vi "RT Init.vi"(8 "error in":errorcluster, 10 "Input Channels":T5[](array[typedef]) format="%.0x", 11 "Custom Device Ref in":T5 format="%.0x") -> (0 "error out":errorcluster, 3 "RT Configuration Data":T1 {"Cal Types" items=["J", "K", "T", "E", "N", "B", "R", "S"]; "Temperature Units" items=["Celcius", "Fahrenheit", "Kelvin", "Rankine"]; "TC Channel Config"."Temperature Units" items=["Celcius", "Fahrenheit", "Kelvin", "Rankine", "Volts"]; "TC Channel Config"."Thermocouple Type" items=["J", "K", "T", "E", "N", "B", "R", "S", "Raw Voltage"]})   [LabVIEW 2011, in "Simulated Thermocouple Custom Device.lvlib"]
uses:
  Simulated Thermocouple Custom Device.lvlib
  <vilib>/NI Veristand/Custom Device API/Custom Device Item Ref.ctl
  RT Config Data.ctl
  TC Channel Config Data.ctl
  TC Selector.ctl
  TC Unit Selector.ctl
  Device Settings.ctl
  Calibration Config Data.ctl
  VO Channel Config Data.ctl
  <vilib>/NI Veristand/Custom Device API/Get Item Property (Variant).vi
  <vilib>/NI Veristand/Custom Device API/Get Item Property (String).vi
  <vilib>/DAQmx/create/channels.llb/DAQmx Create Channel (AO-Voltage-Basic).vi
  <vilib>/DAQmx/create/channels.llb/DAQmx Create Channel (AO-Current-Basic).vi
  <vilib>/NI Veristand/Custom Device API/Custom Device API.lvlib
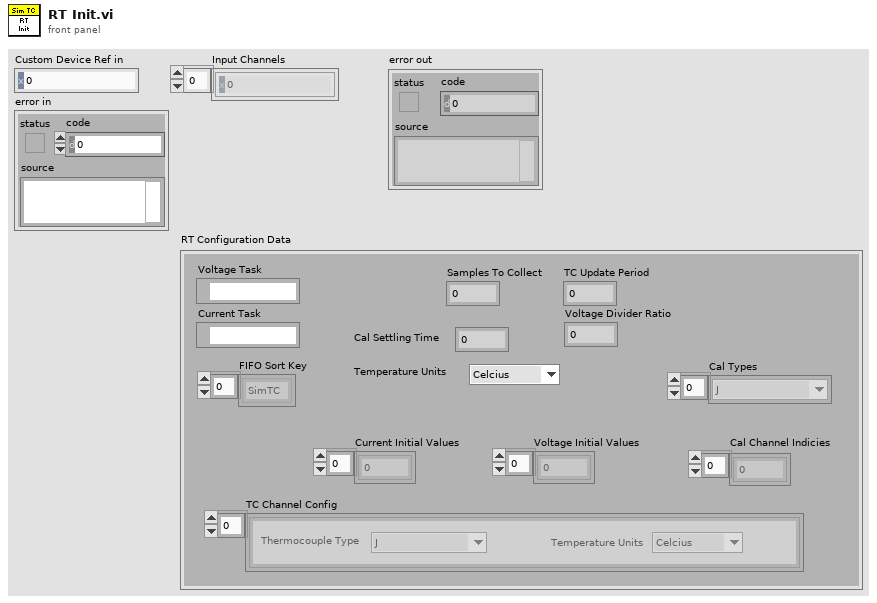
[diagram p1: front panel]
types:
  T1 = typedef "Simulated Thermocouple Custom Device.lvlib/RT Config Data.ctl" = cluster{"Current Task":refnum<k21>, "Voltage Task":refnum<k21>, "FIFO Sort Key":enum16{"SimTC", "Calibration", "VO", "CO"}[], "Cal Channel Indicies":i32[], "Current Initial Values":dbl[], "Voltage Initial Values":dbl[], "TC Channel Config":T2[], "TC Update Period":dbl, "Voltage Divider Ratio":dbl, "Samples To Collect":dbl, "Temperature Units":T4, "Cal Settling Time":dbl, "Cal Types":T3[]}
  T2 = typedef "Simulated Thermocouple Custom Device.lvlib/TC Channel Config Data.ctl" = cluster{"Thermocouple Type":T3, "Temperature Units":T4}
  T3 = typedef "Simulated Thermocouple Custom Device.lvlib/TC Selector.ctl" = u16
  T4 = typedef "Simulated Thermocouple Custom Device.lvlib/TC Unit Selector.ctl" = u16
  T5 = typedef "Custom Device API.lvlib/Custom Device Item Ref.ctl" = u64
  T6 = typedef "Simulated Thermocouple Custom Device.lvlib/Device Settings.ctl" = cluster{"High Side Resistance (Ohms)":dbl, "Low Side Resistance (Ohms)":dbl, "Temperature Units":T4, "Update Rate":dbl, "Physical Device Name":string, "Device Channel Count":u32}
  T7 = typedef "Simulated Thermocouple Custom Device.lvlib/Calibration Config Data.ctl" = cluster{"Local SimTC Chan":string, "Samples To Collect":dbl, "Cal Channel TC Type":T3, "Cal Step Settling Time":dbl}
  T8 = typedef "Custom Device API.lvlib/Custom Device Item Info.ctl" = cluster{"Name":string, "Is Channel":bool, "GUID":string}
  T9 = typedef "Simulated Thermocouple Custom Device.lvlib/VO Channel Config Data.ctl" = cluster{"Initial Value":dbl, "Range Min":dbl, "Range Max":dbl}
  T10 = cluster{"Initial Value":dbl, "Range Min":dbl, "Range Max":dbl}
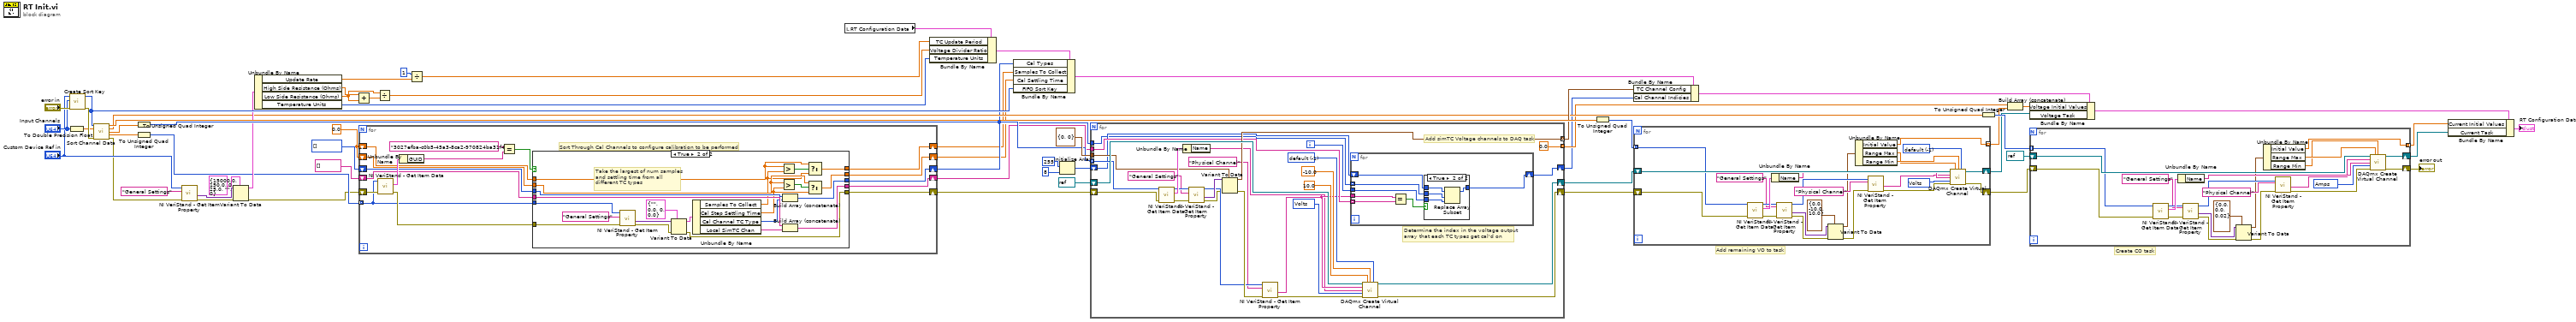
[diagram p0: block diagram]
diagram:
  w9 = T3[] [] items=["J", "K", "T", "E", "N", "B", "R", "S"]
  w13 = 0.0
  # "Create CO task"
  # "Add remaining VO to task"
  n1 = call "Create Sort Key.vi"("error in (no error)"="error in", "Input Channels"="Input Channels", "Custom Device Ref in"="Custom Device Ref in") -> ("error out"=w60:errorcluster, "Key"=w38:enum16{"SimTC", "Calibration", "VO", "CO"}[])  [unwired: 7 in]
  n2 = To Double Precision Float(number="Input Channels") -> (double precision float=w59:dbl[])
  n3 = call "Sort Channel Data.vi"("Key"=w38, "Input Data"=w59, "error in (no error)"=w60) -> ("VO Channels"=w55:dbl[], "CO Channels"=w6:dbl[], "SimTC Channels"=w56:dbl[], "Calibration Channels"=w18:dbl[], "error out"=w19:errorcluster)  [unwired: 8 in]
  n4 = To Unsigned Quad Integer(1:w56) -> (0:w37:u64[])
  n5 = To Unsigned Quad Integer(1:w18) -> (0:w17:u64[])
  n6 = call-poly <vilib>:"NI VeriStand - Get Item Property.vi"("error in (no error)"=w19, "Property Name"="General Settings", "Item Ref in"="Custom Device Ref in") -> ("error out"=w36:errorcluster, "Value"=w34:variant)  [unwired: 5 in, 2 out]
  n7 = Variant To Data(error in=w36, type=T6 {"High Side Resistance (Ohms)"=15000.0, "Low Side Resistance (Ohms)"=150.0, "Temperature Units"=0, "Update Rate"=25.0, "Physical Device Name"="", "Device Channel Count"=0} ("General Settings"), Variant=w34) -> (data=w33:T6, error out=w11:errorcluster)
  n8 = Unbundle By Name(w33) -> ("Update Rate"=w31:dbl, "High Side Resistance (Ohms)"=w30:dbl, "Low Side Resistance (Ohms)"=w29:dbl, "Temperature Units"=w12:T4)
  n9 = Add(x=w30, y=w29) -> (x+y=w28:dbl)
  n10 = for {
    tunnel: w17 -> [w62] mode=indexing
    shift-right: [w70] -> w1
    shift-left: w13 -> [w72]
    shift-right: [w71] -> w2
    shift-left: w13 -> [w73]
    shift-right: [w74] -> w7
    shift-left: string[] [] -> [w68]
    shift-right: [w65] -> w10
    shift-left: w11 -> [w67]
    shift-right: [w63] -> w3
    shift-left: w9 -> [w64]
    # "Sort Through Cal Channels to configure calibration to be performed"
    n11 = call <vilib>:"NI VeriStand - Get Item Data.vi"("error in (no error)"=w67, "Item Ref in"=w62) -> ("error out"=w66:errorcluster, "Item Info"=w77:T8)  [unwired: 6 in, 2 out]
    n12 = Unbundle By Name(w77) -> ("GUID"=w76:string)
    n13 = Equal?(x="3027efba-c0b5-45a3-8ca2-970824ba31f4" ("TC Calibration Config"), y=w76) -> (x = y?=w69:bool)
    n14 = case shown="True" w69 {
      tunnel: w62 -> [_ w103]
      tunnel: [w80 w93] -> w74
      tunnel: w73 -> [w82 w92]
      tunnel: w72 -> [w81 w91]
      tunnel: [w82 w97] -> w71
      tunnel: [w81 w96] -> w70
      tunnel: w68 -> [w80 w94]
      tunnel: w66 -> [w79 w90]
      tunnel: [w79 w89] -> w65
      tunnel: w64 -> [w78 w88]
      tunnel: [w78 w87] -> w63
      frame False {
      }
      frame True {
        # "Take the largest of num samples\nand settling time from all \ndifferent TC types"
        n15 = call-poly <vilib>:"NI VeriStand - Get Item Property.vi"("error in (no error)"=w90, "Property Name"="General Settings", "Item Ref in"=w103) -> ("error out"=w101:errorcluster, "Value"=w100:variant)  [unwired: 5 in, 2 out]
        n16 = Variant To Data(error in=w101, type=T7 {"Local SimTC Chan"="", "Samples To Collect"=0.0, "Cal Channel TC Type"=0, "Cal Step Settling Time"=0.0} ("Cal Info"), Variant=w100) -> (data=w95:T7, error out=w89:errorcluster)
        n17 = Unbundle By Name(w95) -> ("Samples To Collect"=w85:dbl, "Cal Step Settling Time"=w86:dbl, "Cal Channel TC Type"=w83:T3, "Local SimTC Chan"=w84:string)
        n18 = Greater?(x=w92, y=w85) -> (0:w99:bool)
        n19 = Greater?(x=w91, y=w86) -> (0:w98:bool)
        n20 = Build Array (concatenate)(w88, w83) -> (w87:T3[])
        n21 = Build Array (concatenate)(w94, w84) -> (w93:string[])
        n22 = Select(t=w92, s=w99, f=w85) -> (s? t:f=w97:dbl)
        n23 = Select(t=w91, s=w98, f=w86) -> (s? t:f=w96:dbl)
      }
    }
  }
  n24 = Divide(x=w29, y=w28) -> (x/y=w26:dbl)
  n25 = Divide(x=1, y=w31) -> (x/y=w25:dbl)
  n26 = local read "RT Configuration Data"() -> (w27:T1)
  n27 = Bundle By Name(cluster=w27, "TC Update Period"=w25, "Voltage Divider Ratio"=w26, "Temperature Units"=w12) -> (w24:T1)
  n28 = Bundle By Name(cluster=w24, "Cal Types"=w3, "Samples To Collect"=w2, "Cal Settling Time"=w1, "FIFO Sort Key"=w38) -> (w46:T1)
  n29 = Initialize Array(255 ("element"), 8 ("dimension size")) -> (w14:i32[])
  n30 = for {
    shift-right: [w132] -> w52
    shift-left: refnum<k21> refnum ("task in") -> [w133]
    tunnel: w37 -> [w127] mode=indexing
    shift-right: [w114] -> w53
    shift-left: w10 -> [w124]
    tunnel: [w117] -> w45 mode=indexing
    tunnel: T2 {"Thermocouple Type"=0, "Temperature Units"=0} ("TC Channel Config") -> [w116]
    tunnel: [0.0] -> w5 mode=indexing
    tunnel: w7 -> [w112]
    shift-right: [w109] -> w4
    shift-left: w14 -> [w110]
    tunnel: w3 -> [w106]
    i -> [w111]
    w128 = 10348 items=["Volts"=10348, "From Custom Scale"=10065] ("units")
    w129 = -1 items=["default"=-1, "RSE"=10083, "NRSE"=10078, "Differential"=10106, "Pseudodifferential"=12529] ("input terminal configuration")
    # "Add simTC Voltage channels to DAQ task"
    # "Determine the index in the voltage output\narray that each TC types get cal'd on"
    n31 = call <vilib>:"NI VeriStand - Get Item Data.vi"("error in (no error)"=w124, "Item Ref in"=w127) -> ("error out"=w122:errorcluster, "Item Info"=w126:T8, "Item Ref out"=w123:T5)  [unwired: 6 in, 1 out]
    n32 = Unbundle By Name(w126) -> ("Name"=w105:string)
    n33 = call-poly <vilib>:"NI VeriStand - Get Item Property.vi"("error in (no error)"=w122, "Property Name"="General Settings", "Item Ref in"=w123) -> ("error out"=w118:errorcluster, "Value"=w120:variant, "Item Ref out"=w119:T5)  [unwired: 5 in, 1 out]
    n34 = Variant To Data(error in=w118, type=w116, Variant=w120) -> (data=w117:T2, error out=w121:errorcluster)
    n35 = call-poly <vilib>:"NI VeriStand - Get Item Property.vi"("error in (no error)"=w121, "Property Name"="Physical Channel", "Item Ref in"=w119) -> ("error out"=w125:errorcluster, "Value"=w107:string)  [unwired: 5 in, 2 out]
    n36 = for {
      tunnel: w107 -> [w136]
      tunnel: w112 -> [w135] mode=indexing
      tunnel: w111 -> [w139]
      shift-right: [w138] -> w109
      shift-left: w110 -> [w140]
      tunnel: w106 -> [w134] mode=indexing
      n37 = Equal?(x=w136, y=w135) -> (x = y?=w137:bool)
      n38 = case shown="True" w137 {
        tunnel: w134 -> [_ w145]
        tunnel: w140 -> [w141 w144]
        tunnel: w139 -> [_ w143]
        tunnel: [w141 w142] -> w138
        frame False {
        }
        frame True {
          n39 = Replace Array Subset(array=w144, new element=w143, index=w145) -> (w142:i32[])
        }
      }
    }
    n40 = call-poly <vilib>:"DAQmx Create Virtual Channel.vi"("task in"=w133, "maximum value"=10.0, "minimum value"=-10.0, "output terminal configuration"=w129, "physical channels"=w107, "name to assign"=w105, "units"=w128, "error in"=w125) -> ("task out"=w132:refnum<k21>, "error out"=w114:errorcluster)  [unwired: 6 in]
  }
  n41 = To Unsigned Quad Integer(1:w55) -> (0:w54:u64[])
  n42 = Bundle By Name(cluster=w46, "TC Channel Config"=w45, "Cal Channel Indicies"=w4) -> (w43:T1)
  n43 = for {
    shift-right: [w168] -> w44
    shift-left: w52 -> [w169]
    tunnel: w54 -> [w164] mode=indexing
    shift-right: [w150] -> w51
    shift-left: w53 -> [w160]
    tunnel: [w149] -> w23 mode=indexing
    w166 = 10348 items=["Volts"=10348, "From Custom Scale"=10065] ("units")
    w167 = -1 items=["default"=-1, "RSE"=10083, "NRSE"=10078, "Differential"=10106, "Pseudodifferential"=12529] ("input terminal configuration")
    n44 = call <vilib>:"NI VeriStand - Get Item Data.vi"("error in (no error)"=w160, "Item Ref in"=w164) -> ("error out"=w156:errorcluster, "Item Info"=w163:T8, "Item Ref out"=w159:T5)  [unwired: 6 in, 1 out]
    n45 = Unbundle By Name(w163) -> ("Name"=w162:string)
    n46 = call-poly <vilib>:"NI VeriStand - Get Item Property.vi"("error in (no error)"=w156, "Property Name"="General Settings", "Item Ref in"=w159) -> ("error out"=w155:errorcluster, "Value"=w153:variant, "Item Ref out"=w158:T5)  [unwired: 5 in, 1 out]
    n47 = Variant To Data(error in=w155, type=T9 {"Initial Value"=0.0, "Range Min"=-10.0, "Range Max"=10.0} ("VO Channel Config"), Variant=w153) -> (data=w151:T9, error out=w154:errorcluster)
    n48 = Unbundle By Name(w151) -> ("Initial Value"=w149:dbl, "Range Max"=w146:dbl, "Range Min"=w147:dbl)
    n49 = call-poly <vilib>:"NI VeriStand - Get Item Property.vi"("error in (no error)"=w154, "Property Name"="Physical Channel", "Item Ref in"=w158) -> ("error out"=w161:errorcluster, "Value"=w148:string)  [unwired: 5 in, 2 out]
    n50 = call-poly <vilib>:"DAQmx Create Virtual Channel.vi"("task in"=w169, "maximum value"=w146, "minimum value"=w147, "output terminal configuration"=w167, "physical channels"=w148, "name to assign"=w162, "units"=w166, "error in"=w161) -> ("task out"=w168:refnum<k21>, "error out"=w150:errorcluster)  [unwired: 6 in]
  }
  n51 = To Unsigned Quad Integer(1:w6) -> (0:w48:u64[])
  n52 = Build Array (concatenate)(w5, w23) -> (w22:dbl[])
  n53 = Bundle By Name(cluster=w43, "Voltage Initial Values"=w22, "Voltage Task"=w44) -> (w41:T1)
  n54 = for {
    shift-right: [w191] -> w39
    shift-left: refnum<k21> refnum ("task in") -> [w192]
    shift-right: [w177] -> w49
    shift-left: w51 -> [w175]
    tunnel: w48 -> [w176] mode=indexing
    tunnel: [w174] -> w40 mode=indexing
    w173 = 10342 items=["Amps"=10342, "From Custom Scale"=10065] ("units")
    n55 = call <vilib>:"NI VeriStand - Get Item Data.vi"("error in (no error)"=w175, "Item Ref in"=w176) -> ("error out"=w183:errorcluster, "Item Info"=w189:T8, "Item Ref out"=w186:T5)  [unwired: 6 in, 1 out]
    n56 = Unbundle By Name(w189) -> ("Name"=w188:string)
    n57 = call-poly <vilib>:"NI VeriStand - Get Item Property.vi"("error in (no error)"=w183, "Property Name"="General Settings", "Item Ref in"=w186) -> ("error out"=w182:errorcluster, "Value"=w180:variant, "Item Ref out"=w185:T5)  [unwired: 5 in, 1 out]
    n58 = Variant To Data(error in=w182, type=T10 {"Initial Value"=0.0, "Range Min"=0.0, "Range Max"=0.02} ("CO Channel Config"), Variant=w180) -> (data=w179:T10, error out=w181:errorcluster)
    n59 = Unbundle By Name(w179) -> ("Initial Value"=w174:dbl, "Range Max"=w171:dbl, "Range Min"=w170:dbl)
    n60 = call-poly <vilib>:"NI VeriStand - Get Item Property.vi"("error in (no error)"=w181, "Property Name"="Physical Channel", "Item Ref in"=w185) -> ("error out"=w187:errorcluster, "Value"=w172:string)  [unwired: 5 in, 2 out]
    n61 = call-poly <vilib>:"DAQmx Create Virtual Channel.vi"("task in"=w192, "maximum value"=w171, "minimum value"=w170, "physical channels"=w172, "name to assign"=w188, "units"=w173, "error in"=w187) -> ("task out"=w191:refnum<k21>, "error out"=w177:errorcluster)  [unwired: 7 in]
  }
  "error out" <- w49
  n62 = Bundle By Name(cluster=w41, "Current Initial Values"=w40, "Current Task"=w39) -> (→"RT Configuration Data":T1)
